vi "GetGateMeasAlmMode.vi"(8 "错误输入（无错误）":errorcluster, 11 "通道闸门序号":i32) -> (0 "错误输出":errorcluster, 3 "返回值":u16)   [LabVIEW 2014]
uses:
  ZXUTConfigMgr.dll
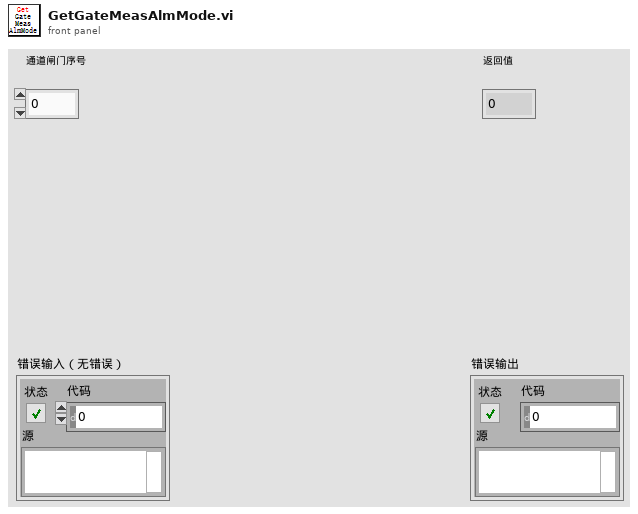
[diagram p1: front panel]
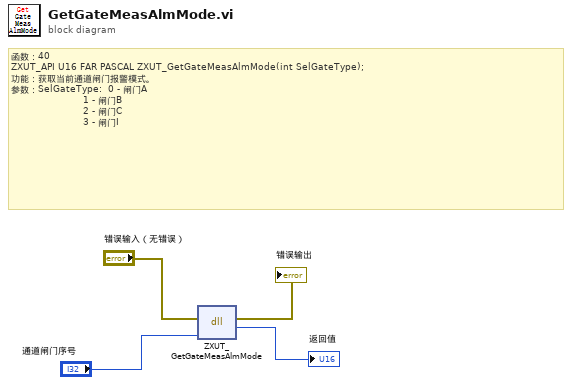
[diagram p0: block diagram]
diagram:
  # "函数：40\nZXUT_API U16\tFAR PASCAL ZXUT_GetGateMeasAlmMode(int SelGateType);\n功能：获取当前通道闸门报警模式。\n参数：SelGateType:  0 - 闸门A \n                        1 - 闸门B\n                        2 - 闸门C\n                        3 - 闸门I"
  n1 = dll-call lib="PTH2eabs D软件超声实时监测软件ZXUTAppDemo(华南理工V02.00)X86DllZXUTConfigMgr.dll" fn="ZXUT_GetGateMeasAlmMode"(error in="错误输入（无错误）", "SelGateType"="通道闸门序号") -> (error out=→"错误输出":errorcluster, "返回值"=→"返回值":u16)  [unwired: 3 in, 1 out]
